vi "setEventRaiseMirrorComplete.vi"(10 "EventRaiseMirrorComplete":refnum<user-event>, 11 "UserEvents in":refnum<class "UserEvents.lvclass">) -> (3 "UserEvents out":refnum<class "UserEvents.lvclass">)   [LabVIEW 2016, in "UserEvents.lvclass"]
uses:
  UserEvents.lvclass
  DataTypes/Topics/EventRaiseMirrorComplete.ctl
  DataTypes/Topics/Parts/Timestamp.ctl
  UserEvents.lvclass/UserEvents.ctl
  DataTypes/Topics/M1M3SupportTopics.lvlib
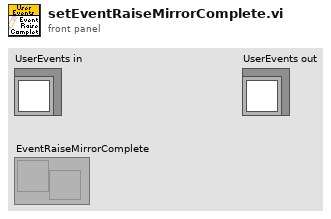
[diagram p1: front panel]
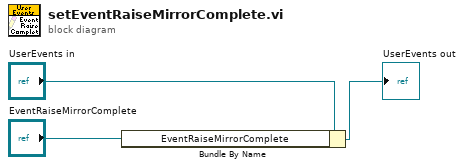
[diagram p0: block diagram]
diagram:
  n1 = Bundle By Name(cluster="UserEvents in", "EventRaiseMirrorComplete"="EventRaiseMirrorComplete") -> (→"UserEvents out":refnum<class "UserEvents.lvclass">)
